vi "Auto Number Query.vi"(8 "error in (no error)":errorcluster, 10 "Query":string="SELECT * FROM AUTO NUMBER WHERE [sModelNumebr] is NULL;", 11 "Connection Refnum":T2) -> (0 "error out":errorcluster, 2 "Auto Number Records":T1[](array[typedef]), 3 "Connection Refnum":T2, 4 "Data Present?":bool)   [LabVIEW 2011]
uses:
  Summitek EXT/ODBC/SQL Controls/Connection Refnum.ctl
  Auto Number Record.ctl
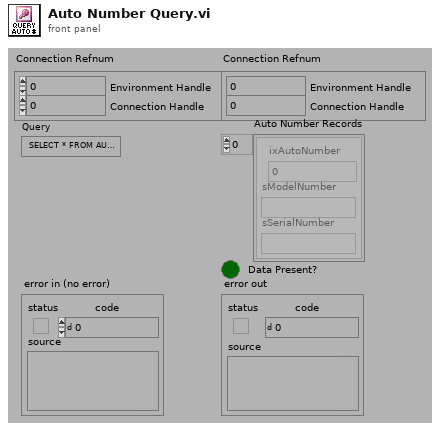
[diagram p1: front panel]
types:
  T1 = typedef "Auto Number Record.ctl" = cluster{"ixAutoNumber":i32, "sModelNumber":string, "sSerialNumber":string}
  T2 = typedef "Connection Refnum.ctl" = cluster{"Environment Handle":i32, "Connection Handle":i32}
  T3 = typedef "Statement Refnum.ctl" = cluster{"Statement Handle":i32, "Parameter Number":u16}
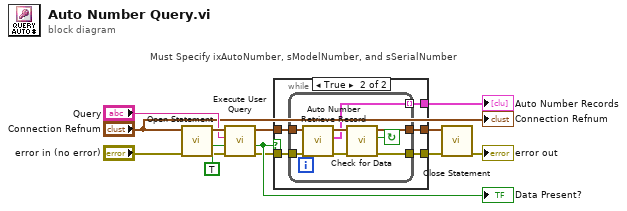
[diagram p0: block diagram]
diagram:
  # "Must Specify ixAutoNumber, sModelNumber, and sSerialNumber"
  n1 = call "Open Statement.vi"("error in (no error)"="error in (no error)", "Connection Refnum"="Connection Refnum") -> ("error out"=w8:errorcluster, "Statement Refnum"=w9:T3)  [unwired: 4 out]
  n2 = call "Execute User Query.vi"("error in (no error)"=w8, "Return Data? (f)"=TRUE, "User Query"="Query", "Statement Refnum"=w9) -> ("error out"=w12:errorcluster, "Data Present?"=w13:bool, "Statement Refnum"=w11:T3)  [unwired: 1 out]
  "Data Present?" <- w13
  n3 = case shown="True" w13 {
    tunnel: w12 -> [w14 w19]
    tunnel: w11 -> [w15 w20]
    tunnel: [w14 w17] -> w7
    tunnel: [w15 w18] -> w6
    tunnel: [_ w16] -> w3
    frame False {
    }
    frame True {
      n4 = while {
        tunnel: w20 -> [w27]
        tunnel: w19 -> [w26]
        tunnel: [w24] -> w18
        tunnel: [w22] -> w17
        tunnel: [w21] -> w16 mode=indexing
        stop <- w28 continue-if-true
        n5 = call "Auto Number Retrieve Record.vi"("error in (no error)"=w26, "Statement Refnum"=w27) -> ("error out"=w23:errorcluster, "Auto Number Record"=w21:T1, "Statement Refnum"=w25:T3)  [unwired: 1 in, 6 out]
        n6 = call "Check for Data.vi"("error in (no error)"=w23, "Statement Refnum"=w25) -> ("error out"=w22:errorcluster, "Data Present?"=w28:bool, "Statement Refnum"=w24:T3)  [unwired: 3 out]
      }
    }
  }
  "Auto Number Records" <- w3
  n7 = call "Close Statement.vi"("error in (no error)"=w7, "Statement Refnum"=w6) -> ("error out"=→"error out":errorcluster)  [unwired: 5 out]
  "Connection Refnum" <- "Connection Refnum"
